vi "PythonSession.vi"(6 "PythonPath":path, 7 "SessionName":string, 8 "error in (no error)":errorcluster, 11 "PythonVersion":string) -> (0 "error out":errorcluster, 3 "PythonSession":refnum<class "PythonSession.lvclass">)   [LabVIEW 2022 SP3, in "PythonWrapper.lvlib" / "PythonSession.lvclass"]
uses:
  PythonSession.lvclass
  PythonSession.lvclass/PythonSession.ctl
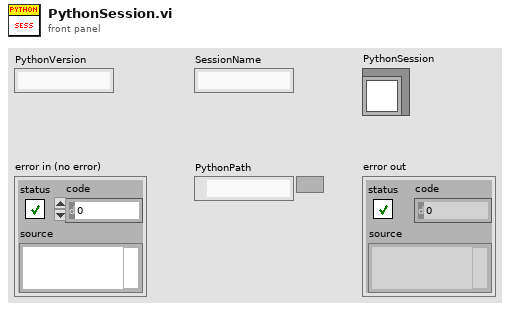
[diagram p1: front panel]
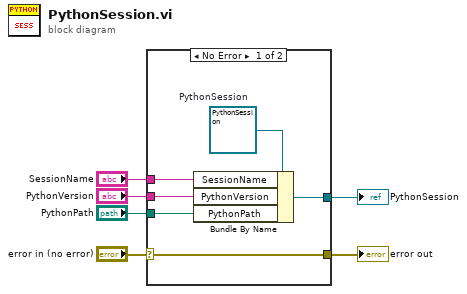
[diagram p0: block diagram]
diagram:
  n1 = case shown="No Error" "error in (no error)" {
    selector: "error in (no error)" -> [w11 w13]
    tunnel: [w11 w13] -> w5
    tunnel: [w7 _] -> w4
    tunnel: "PythonVersion" -> [w9 _]
    tunnel: "PythonPath" -> [w8 _]
    tunnel: "SessionName" -> [w10 _]
    frame No Error {
      w12 = refnum<class "PythonSession.lvclass"> refnum  # PythonSession
      n2 = Bundle By Name(cluster=w12, "SessionName"=w10, "PythonVersion"=w9, "PythonPath"=w8) -> (w7:refnum<class "PythonSession.lvclass">)
    }
    frame Error {
    }
  }
  "error out" <- w5
  "PythonSession" <- w4
